vi "AR.vi"(11 "Trigger":bool) -> (7 "Sample Out":fxp<+,8,0>)   [LabVIEW 2015]
doc: "Eliminates Decay and Sustain phases and narrows down the ADSR envelope to a simple Attack-Release evolution."
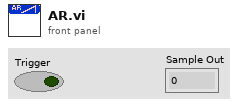
[diagram p1: front panel]
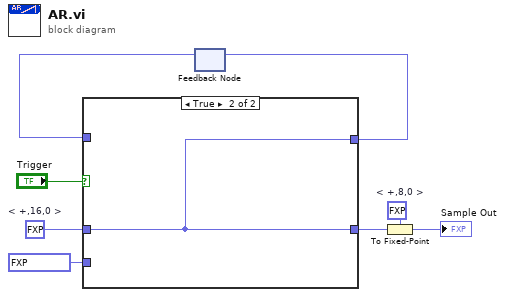
[diagram p0: block diagram]
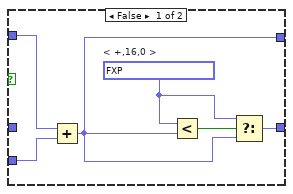
[diagram p2: hidden frame]
diagram:
  w4 = fxp<+,8,0> 0.0  # < +,8,0 >
  w6 = fxp<+,16,0> 0.0  # < +,16,0 >
  n1 = feedback #1() -> (w2:fxp<+,16,0>)  [unwired: 1 in]
  n2 = case shown="True" "Trigger" {
    tunnel: w6 -> [_ w15]
    tunnel: fxp<+,16,0> 1.52587890625e-05 ("1/Attack") -> [w14 _]
    tunnel: [w10 w15] -> w3
    tunnel: w2 -> [w13 _]
    tunnel: [w11 w15] -> w5
    frame False {
      w9 = fxp<+,16,0> 0.9999847412109375  # < +,16,0 >
      n3 = Add(x=w13, y=w14) -> (x+y=w10:fxp<+,16,0>)
      n4 = Less?(x=w9, y=w10) -> (x < y?=w12:bool)
      n5 = Select(t=w9, s=w12, f=w10) -> (s? t:f=w11:fxp<+,16,0>)
    }
    frame True {
    }
  }
  n6 = feedback-in #1(w3) -> ()
  n7 = To Fixed-Point(fixed-point type=w4, number=w5) -> (fixed-point=→"Sample Out":fxp<+,8,0>)
